vi "Read Profibus initiate data.vi"(8 "error in (no error)":errorcluster, 11 "Profibus in":refnum<class "Profibus.lvclass">) -> (0 "error out":errorcluster, 2 "Initiate data":T1={"Communication ref.:"=1, "Send timeout:"=0, "Feat. supp. 1:"=1, "Feat. supp. 2:"=0, "Profile feat. supp. 1:"=0, "Profile feat. supp. 2:"=0, "Profile ID number:"=0, "Addional address parameter"={"S-Type"=FALSE, "S-Length:"=2, "D-Type"=FALSE, "D-Length:"=2, "Data:"=[0, 0, 0, 0]}} {"Addional address parameter"."D-Length:" format="%0.0f"; "Addional address parameter"."S-Length:" format="%0.0f"; "Addional address parameter"."Data:" format="%.0x"; "Feat. supp. 2:" format="%.0x"; "Feat. supp. 1:" format="%.0x"; "Profile feat. supp. 2:" format="%.0x"; "Profile feat. supp. 1:" format="%.0x"; "Profile ID number:" format="%.0x"; "Send timeout:" format="%0.0f"; "Communication ref.:" min=1 max=49 format="%0.0f"}, 3 "Profibus out":refnum<class "Profibus.lvclass">)   [LabVIEW 2016, in "Profibus.lvclass"]
uses:
  Profibus.lvclass
  Profibus VISA Driver/DF PROFI II.llb/CS_PB_DPV1_MSAC2_InitiateReqData.ctl
  Profibus.lvclass/Profibus.ctl
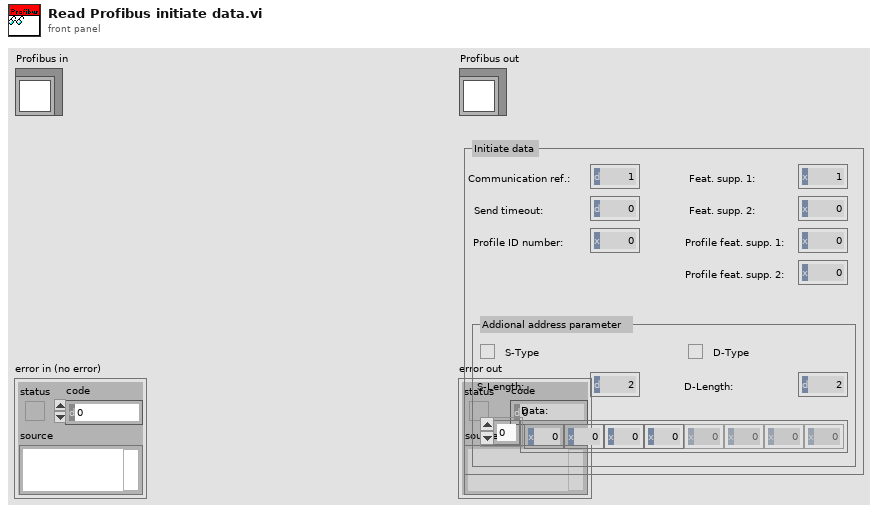
[diagram p1: front panel]
types:
  T1 = typedef "CS_PB_DPV1_MSAC2_InitiateReqData.ctl" = cluster{"Communication ref.:":u8, "Send timeout:":u16, "Feat. supp. 1:":u8, "Feat. supp. 2:":u8, "Profile feat. supp. 1:":u8, "Profile feat. supp. 2:":u8, "Profile ID number:":u16, "Addional address parameter":cluster{"S-Type":bool, "S-Length:":u8, "D-Type":bool, "D-Length:":u8, "Data:":u8[]}}
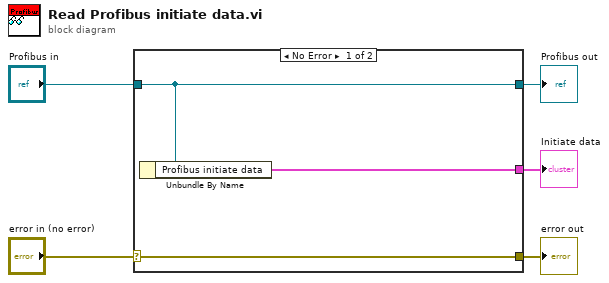
[diagram p0: block diagram]
diagram:
  n1 = case shown="No Error" "error in (no error)" {
    selector: "error in (no error)" -> [w8 w9]
    tunnel: [w8 w9] -> w4
    tunnel: [w7 w10] -> w2
    tunnel: "Profibus in" -> [w7 w10]
    tunnel: [w6 _] -> w1
    frame No Error {
      n2 = Unbundle By Name(w7) -> ("Profibus initiate data"=w6:T1)
    }
    frame Error {
    }
  }
  "error out" <- w4
  "Profibus out" <- w2
  "Initiate data" <- w1
